vi "FTW-JSON-Serialize.vi"(0 "JSON Object":refnum<data-value>, 11 "error in":errorcluster) -> (4 "JSON Object out":refnum<data-value>, 6 "JSON String (UTF-8)":string, 15 "error out":errorcluster)   [LabVIEW 2015]
uses:
  core/FTW-JSON-Core-Structure.ctl
panel:
  # "Inputs"
  # "Outputs"
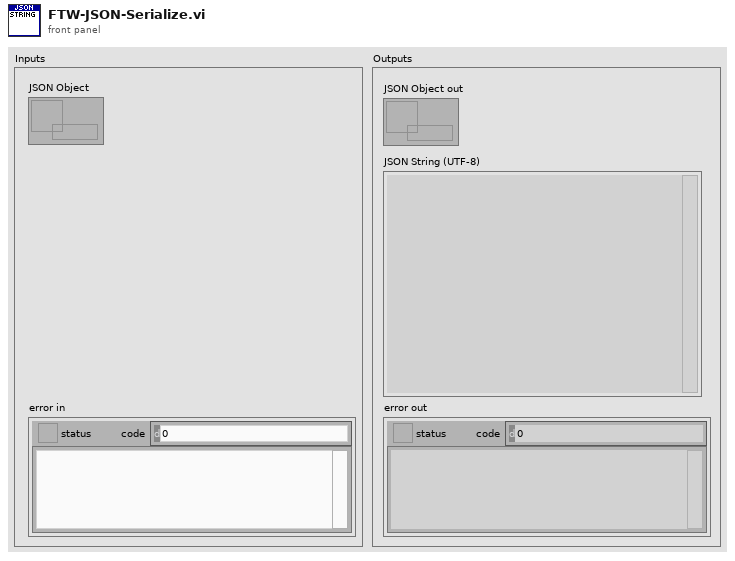
[diagram p1: front panel]
types:
  T1 = typedef "FTW-JSON-Core-Structure.ctl" = cluster{"JSON Object":i64, "Encoding Flags":i64, "Decoding Flags":i64}
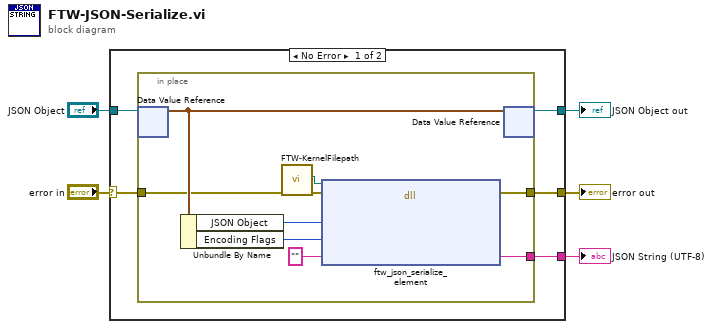
[diagram p0: block diagram]
diagram:
  n1 = case shown="No Error" "error in" {
    selector: "error in" -> [w10 w21]
    tunnel: [w9 w21] -> w5
    tunnel: [w7 w20] -> w3
    tunnel: "JSON Object" -> [w6 w20]
    tunnel: [w8 _] -> w1
    frame No Error {
      n2 = in-place {
        in-place-border: w10 -> [w13]
        in-place-border: [w16] -> w9
        in-place-border: [w17] -> w8
        n3 = in-place-dvr #1(w6) -> (w19:T1)  [unwired: 1 out]
        n4 = Unbundle By Name(w19) -> ("JSON Object"=w15:i64, "Encoding Flags"=w14:i64)
        n5 = call "FTW-KernelFilepath.vi"("error in"=w13) -> ("error out"=w12:errorcluster, "Library Filepath"=w11:path)  [unwired: 8 in, 1 out]
        n6 = dll-call lib="?" fn="ftw_json_serialize_element"(path in=w11, error in=w12, "JSON Object Pointer"=w15, "Flags"=w14, "Serialized String"="") -> (error out=w16:errorcluster, "Serialized String"=w17:string)  [unwired: 4 in, 1 out]
        n7 = in-place-dvr #1(w19) -> (w7:refnum<data-value>)  [unwired: 1 out]
      }
    }
    frame Error {
    }
  }
  "error out" <- w5
  "JSON Object out" <- w3
  "JSON String (UTF-8)" <- w1
